vi "VI Tree.vi"   [LabVIEW 2015, in "Voltech PM1000+.lvlib"]
doc: "This is the instrument driver for the PM1000+ Power Analyzer. The VI Tree displays all the user-callable VIs of the instrument driver in an organized table."
uses:
  <instrlib>/Voltech PM1000+/Voltech PM1000+.lvlib
  <instrlib>/Voltech PM1000+/Public/Configure/Configure Measurements (Normal).vi
panel:
  # "(c) 2008-2009 Voltech Instruments.  ALL RIGHTS RESERVED."
  # "SEE DIAGRAM\nFOR VI TREE."
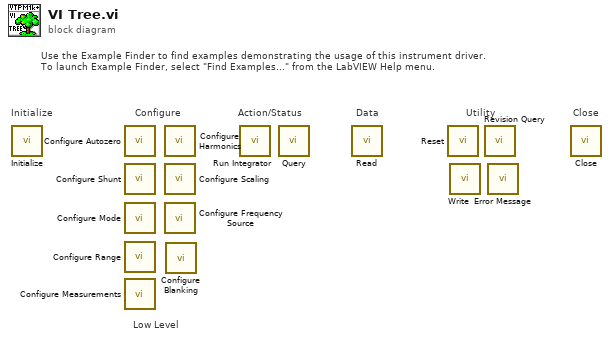
[diagram p0: block diagram]
diagram:
  # "Action/Status"
  # "Low Level"
  # "Use the Example Finder to find examples demonstrating the usage of this instrument driver.\nTo launch Example Finder, select \"Find Examples...\" from the LabVIEW Help menu."
  # "Configure"
  # "Utility"
  # "Data"
  # "Close"
  # "Initialize"
  n1 = call <instrlib>:"Initialize.vi"() -> ()  [unwired: 10 in, 2 out]
  n2 = call <instrlib>:"Configure Autozero.vi"() -> ()  [unwired: 10 in, 2 out]
  n3 = call <instrlib>:"Configure Shunt.vi"() -> ()  [unwired: 10 in, 2 out]
  n4 = call <instrlib>:"Configure Mode.vi"() -> ()  [unwired: 10 in, 2 out]
  n5 = call <instrlib>:"Configure Range.vi"() -> ()  [unwired: 10 in, 2 out]
  n6 = call-poly <instrlib>:"Configure Measurements.vi"() -> ()  [unwired: 10 in, 2 out]
  n7 = call <instrlib>:"Configure Harmonics.vi"() -> ()  [unwired: 10 in, 2 out]
  n8 = call <instrlib>:"Configure Scaling.vi"() -> ()  [unwired: 10 in, 2 out]
  n9 = call <instrlib>:"Configure Frequency Source.vi"() -> ()  [unwired: 10 in, 2 out]
  n10 = call <instrlib>:"Configure Blanking.vi"() -> ()  [unwired: 10 in, 2 out]
  n11 = call <instrlib>:"Run Integrator.vi"() -> ()  [unwired: 10 in, 2 out]
  n12 = call <instrlib>:"Query.vi"() -> ()  [unwired: 9 in, 3 out]
  n13 = call <instrlib>:"Read.vi"() -> ()  [unwired: 9 in, 3 out]
  n14 = call <instrlib>:"Reset.vi"() -> ()  [unwired: 10 in, 2 out]
  n15 = call <instrlib>:"Write.vi"() -> ()  [unwired: 10 in, 2 out]
  n16 = call <instrlib>:"Revision Query.vi"() -> ()  [unwired: 8 in, 4 out]
  n17 = call <instrlib>:"Error Message.vi"() -> ()  [unwired: 14 in, 2 out]
  n18 = call <instrlib>:"Close.vi"() -> ()  [unwired: 11 in, 1 out]
